vi "Test Snake Does Not Move When Not Alive.vi"(8 "error in (no error)":errorcluster, 11 "Test Case In":refnum<class "Snake Test.lvclass">) -> (0 "error out":errorcluster, 3 "Test Case Out":refnum<class "Snake Test.lvclass">)   [LabVIEW 2020, in "Snake Test.lvclass"]
uses:
  Snake Test.lvclass
  C:/Program Files (x86)/National Instruments/LabVIEW 2020/vi.lib/Astemes/LUnit/Test Case.lvclass
  source/Particle/Position.ctl
  source/Snake/Direction.ctl
  <vilib>/Astemes/LUnit/Test Case.lvclass/Test Case.ctl
  <vilib>/Astemes/LUnit/Set Assertion Type.vi
  <vilib>/Astemes/LUnit/Palette/Pass.vi
  <vilib>/Astemes/LUnit/Palette/Fail.vi
  <vilib>/Astemes/LUnit/Add test result.vi
  <vilib>/Astemes/LUnit/LUnit Record Assertion Result.vi
  <vilib>/Astemes/LUnit/LUnit Aggregate Assertion Results.vi
  <vilib>/Astemes/LUnit/Method Result/LUnit Merge Status.vi
  <vilib>/Astemes/LUnit/LUnit Concatenate result strings.vi
  Snake Test.lvclass/Snake Test.ctl
  source/Snake/Snake.lvclass
  source/Particle.lvclass
  <vilib>/Astemes/LUnit/Test Case.lvclass
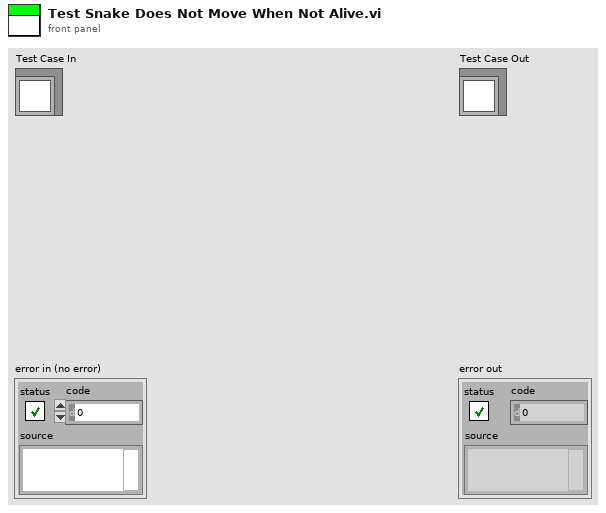
[diagram p1: front panel]
types:
  T1 = typedef "Particle.lvclass/Position.ctl" = cluster{"X":i32, "Y":i32}
  T2 = typedef "Direction.ctl" = enum16{"X", "-X", "Y", "-Y"}
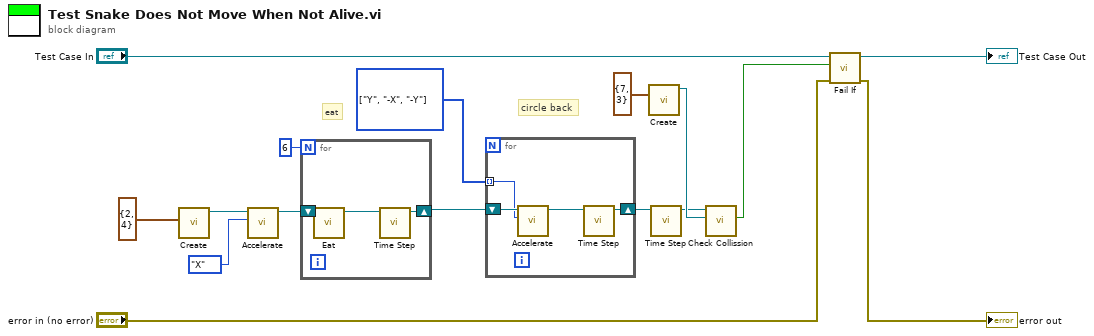
[diagram p0: block diagram]
diagram:
  w7 = T2[] [enum."Y", enum."-X", enum."-Y"] items=["X", "-X", "Y", "-Y"] ("Array")
  # "circle back"
  # "eat"
  n1 = call "Create.vi"("Position"=T1 {"X"=2, "Y"=4}) -> ("Snake out"=w12:refnum<class "Snake.lvclass">)  [unwired: 10 in]
  n2 = call "Accelerate.vi"("Direction"=enum16{"X", "-X", "Y", "-Y"}."X", "Snake in"=w12) -> ("Snake out"=w9:refnum<class "Snake.lvclass">)  [unwired: 9 in]
  n3 = for {
    N: 6 -> [_]
    shift-right: [w18] -> w6
    shift-left: w9 -> [w19]
    n4 = call "Eat.vi"("Snake in"=w19) -> ("Snake out"=w17:refnum<class "Snake.lvclass">)  [unwired: 10 in]
    n5 = call "Time Step.vi"("Snake in"=w17) -> ("Snake out"=w18:refnum<class "Snake.lvclass">)  [unwired: 10 in]
  }
  n6 = for {
    shift-right: [w22] -> w3
    shift-left: w6 -> [w23]
    tunnel: w7 -> [w20] mode=indexing
    n7 = call "Accelerate.vi"("Direction"=w20, "Snake in"=w23) -> ("Snake out"=w21:refnum<class "Snake.lvclass">)  [unwired: 9 in]
    n8 = call "Time Step.vi"("Snake in"=w21) -> ("Snake out"=w22:refnum<class "Snake.lvclass">)  [unwired: 10 in]
  }
  n9 = call "Create.vi"("Position"=T1 {"X"=7, "Y"=3}) -> ("Particle out"=w4:refnum<class "Particle.lvclass">)  [unwired: 10 in]
  n10 = call "Time Step.vi"("Snake in"=w3) -> ("Snake out"=w1:refnum<class "Snake.lvclass">)  [unwired: 10 in]
  n11 = call "Check Collission.vi"("Particle"=w4, "Snake in"=w1) -> ("Collided?"=w2:bool)  [unwired: 8 in, 1 out]
  n12 = call <vilib>:"Fail If.vi"("error in (no error)"="error in (no error)", "Fail?"=w2, "LUnit Test Case In"="Test Case In") -> ("error out"=→"error out":errorcluster, "LUnit Test Case Out"=→"Test Case Out":refnum<class "Snake Test.lvclass">)  [unwired: 7 in]
